vi "IP2 SMF out.vi"() -> ()   [LabVIEW 2020]
panel:
  out "Boolean":bool
  out "No errors =T 2":bool
  out "No errors =T":bool
  out "Numeric 4":dbl=199.0
  in  "SMF Z out position 3":dbl
  out "Numeric 3":dbl=199.0
  in  "DPM Z out position 2":dbl=37.0
  out "Numeric 2":dbl=199.0
  in  "DPM X out position":dbl=107.129
  in  "Debris in position":dbl=199.0
  out "Numeric":dbl=199.0
  # "SMF Out Positions"
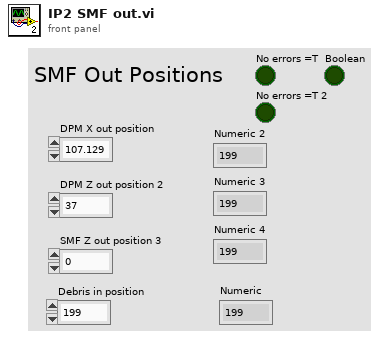
[diagram p1: front panel]
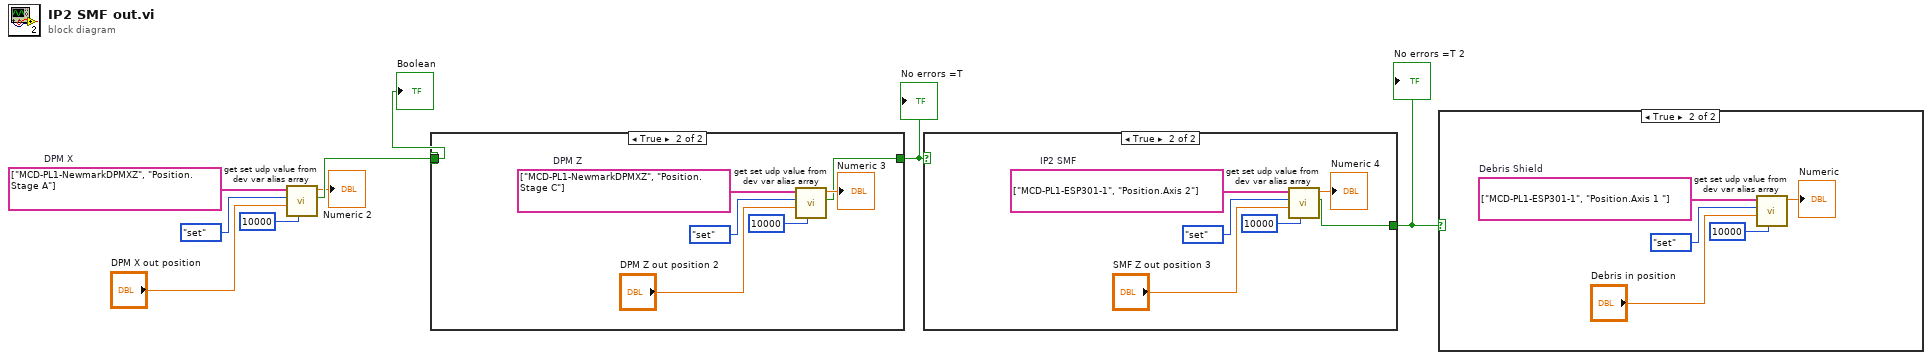
[diagram p0: block diagram]
diagram:
  w6 = string[] ["MCD-PL1-NewmarkDPMXZ", "Position.Stage A"]  # DPM X
  n1 = call "get set udp value from dev var alias array.vi"("slow timeout ms (3000)"=10000, "Set position"="DPM X out position", "get or set"=enum16{"get", "set"}."set", "dev variable alias Motors X"=w6) -> ("No errors =T"=w9:bool, "Numeric"=→"Numeric 2":dbl)  [unwired: 5 in, 1 out]
  n2 = case shown="True" w9 {
    selector: w9 -> [_ w10]
    tunnel: [_ w11] -> w8
    tunnel: [_ w10] -> w1
    frame False {
    }
    frame True {
      w16 = string[] ["MCD-PL1-NewmarkDPMXZ", "Position.Stage C"]  # DPM Z
      n3 = call "get set udp value from dev var alias array.vi"("slow timeout ms (3000)"=10000, "Set position"="DPM Z out position 2", "get or set"=enum16{"get", "set"}."set", "dev variable alias Motors X"=w16) -> ("No errors =T"=w11:bool, "Numeric"=→"Numeric 3":dbl)  [unwired: 5 in, 1 out]
    }
  }
  "No errors =T" <- w8
  "Boolean" <- w1
  n4 = case shown="True" w8 {
    tunnel: [_ w17] -> w7
    frame False {
    }
    frame True {
      w22 = string[] ["MCD-PL1-ESP301-1", "Position.Axis 2"]  # IP2 SMF
      n5 = call "get set udp value from dev var alias array.vi"("slow timeout ms (3000)"=10000, "Set position"="SMF Z out position 3", "get or set"=enum16{"get", "set"}."set", "dev variable alias Motors X"=w22) -> ("No errors =T"=w17:bool, "Numeric"=→"Numeric 4":dbl)  [unwired: 5 in, 1 out]
    }
  }
  "No errors =T 2" <- w7
  n6 = case shown="True" w7 {
    frame False {
    }
    frame True {
      w27 = string[] ["MCD-PL1-ESP301-1", "Position.Axis 1 "]  # Debris Shield
      n7 = call "get set udp value from dev var alias array.vi"("slow timeout ms (3000)"=10000, "Set position"="Debris in position", "get or set"=enum16{"get", "set"}."set", "dev variable alias Motors X"=w27) -> ("Numeric"=→"Numeric":dbl)  [unwired: 5 in, 2 out]
    }
  }
